vi "Main.vi"(8 "error in":errorcluster, 11 "TCP Read in":refnum<class "TCP Read.lvclass">) -> (0 "error out":errorcluster, 3 "TCP Read out":refnum<class "TCP Read.lvclass">)   [LabVIEW 2017, in "_TCP Client.lvlib" / "TCP Read.lvclass"]
doc: "The <b>Queued Message Handler</b> of the Worker that owns this VI."
uses:
  TCP Read.lvclass
  C:/SC/Source Code/VIPM/LabVIEW 20xx/vi.lib/addons/_Workers/Library/Classes/Worker/Worker.lvclass
  Initialization Data.ctl
  Response Cases.ctl
  <vilib>/addons/_Workers/Library/Case Label.ctl
  <vilib>/addons/_Workers/Library/Classes/Message Queue/Message Queue.lvclass
  TCP Read.lvclass/TCP Read.ctl
  rsp_Connection Lost.ctl
  <vilib>/addons/_Workers/Library/Workers.lvlib
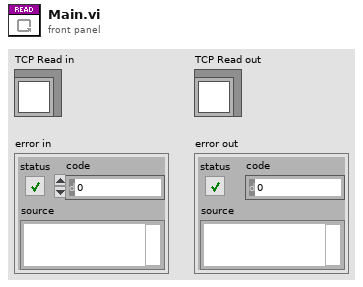
[diagram p1: front panel]
types:
  T1 = typedef "_TCP Client.lvlib/TCP Read.lvclass/Initialization Data.ctl" = cluster{"Response Cases":T2, "Connection ID":refnum<k5>, "Forwarding Queue":refnum<class "Message Queue.lvclass">, "Forwarding Case":T3, "Server Name":string}
  T2 = typedef "_TCP Client.lvlib/TCP Read.lvclass/Response Cases.ctl" = cluster{"Connection Lost":T3}
  T3 = typedef "Workers.lvlib/Case Label.ctl" = string
  T4 = enum16{"Standard", "Buffered", "CRLF", "Immediate"}
  T5 = typedef "_TCP Client.lvlib/TCP Read.lvclass/rsp_Connection Lost.ctl" = cluster{"Connection ID":refnum<k5>, "TCP Read Queue":refnum<class "Message Queue.lvclass">}
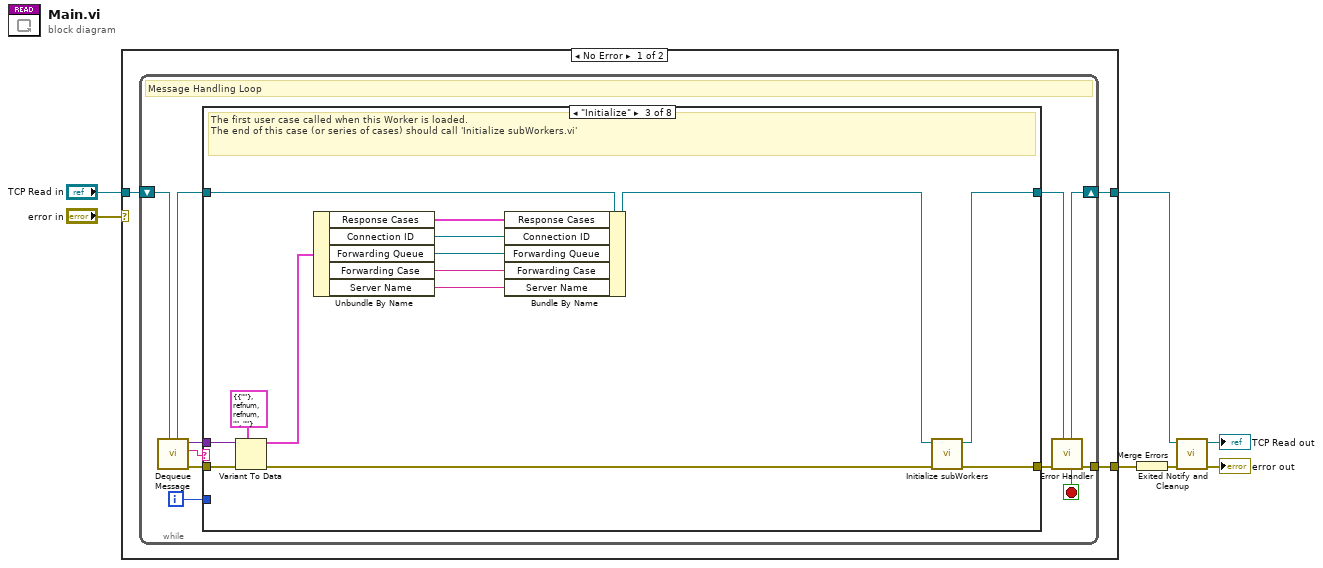
[diagram p0: block diagram]
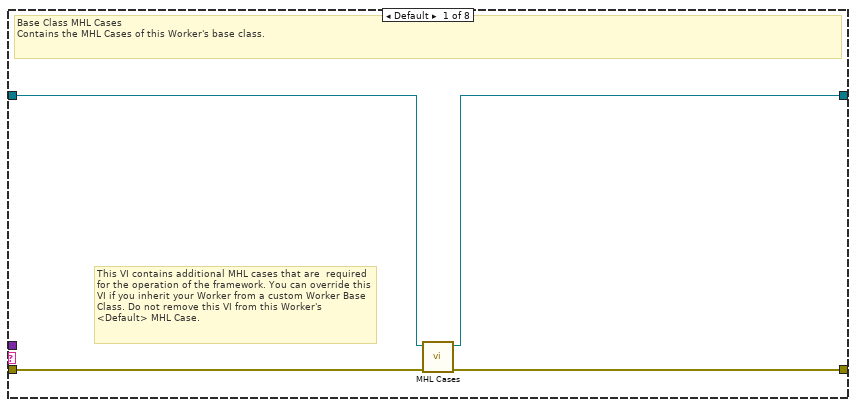
[diagram p2: hidden frame]
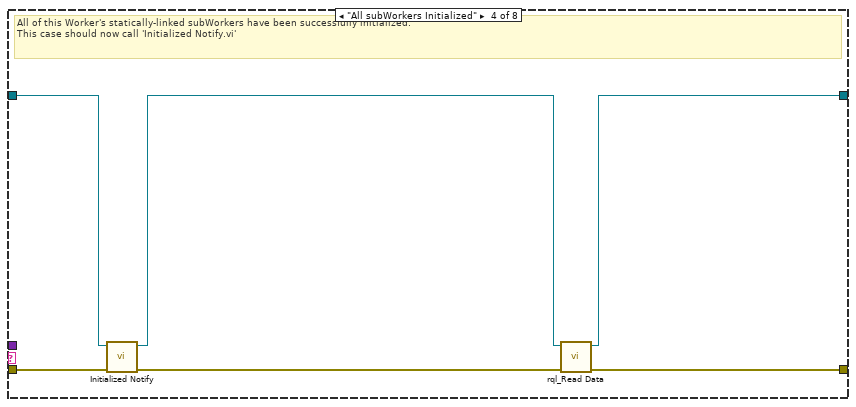
[diagram p4: hidden frame]
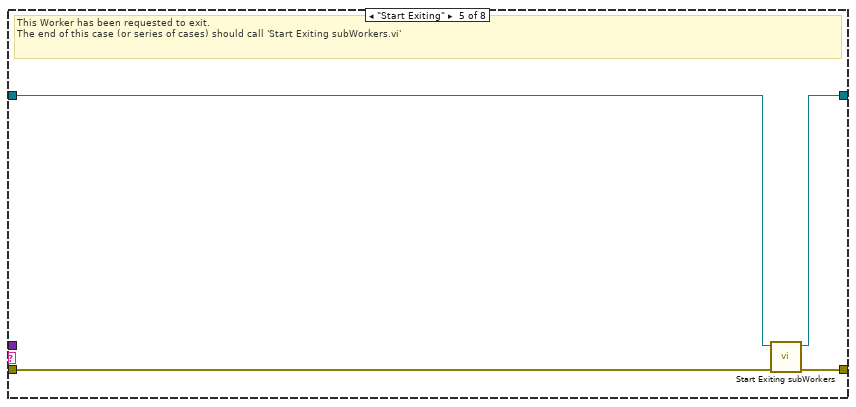
[diagram p5: hidden frame]
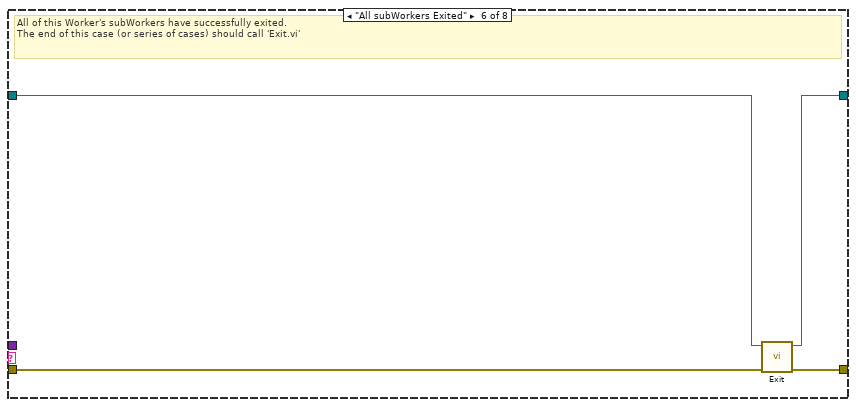
[diagram p6: hidden frame]
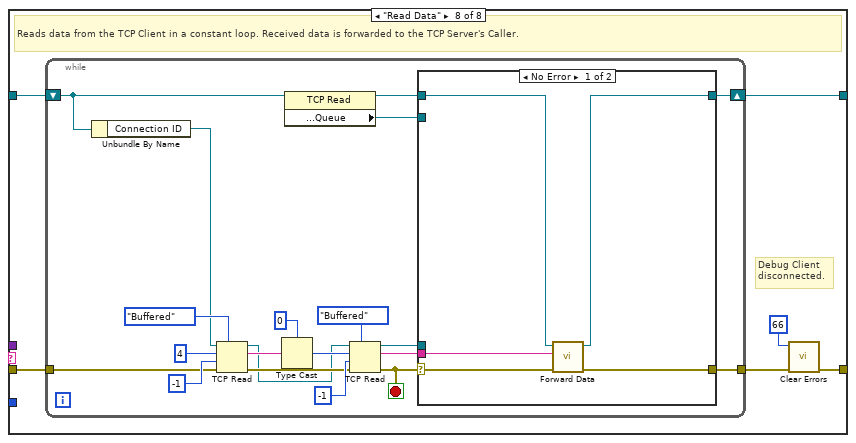
[diagram p8: hidden frame]
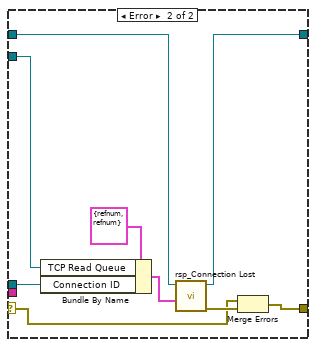
[diagram p9: hidden frame]
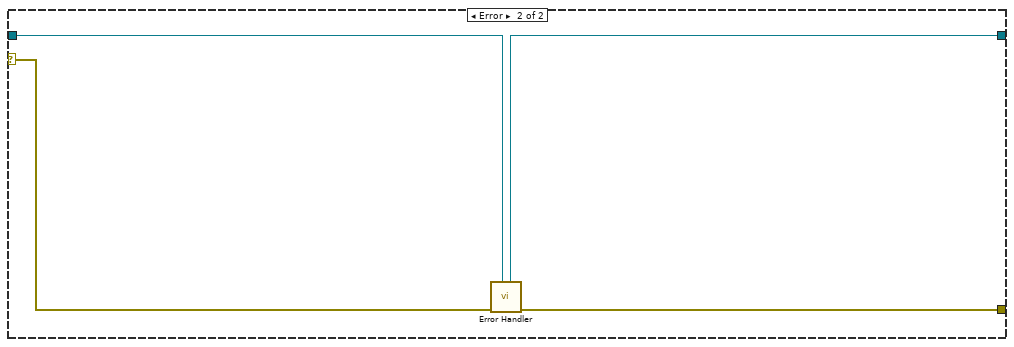
[diagram p10: hidden frame]
diagram:
  n1 = case shown="No Error" "error in" {
    tunnel: "TCP Read in" -> [w8 w99]
    tunnel: [w10 w100] -> w1
    tunnel: [w9 w98] -> w7
    selector: "error in" -> [_ w101]
    frame No Error {
      n2 = while {
        shift-right: [w19] -> w9
        shift-left: w8 -> [w21]
        tunnel: [w20] -> w10
        i -> [w12]
        stop <- w13 stop-if-true
        # "Message Handling Loop"
        n3 = call-dynamic "Dequeue Message.vi"("Worker"=w21) -> ("error out"=w18:errorcluster, "Case out"=w14:string, "Data out"=w11:variant, "Worker out"=w16:refnum<class "TCP Read.lvclass">)  [unwired: 6 in, 1 out]
        n4 = case "Worker MHL Case Structure (DO NOT CHANGE LABEL NAME)" shown="\"Initialize\"" w14 {
          tunnel: w18 -> [w25 w26 w39 w47 w48 w55 w57 w61]
          tunnel: [w24 w26 w41 w44 w51 w54 w57 w58] -> w17
          tunnel: w16 -> [w23 w27 w38 w45 w49 w53 w56 w62]
          tunnel: [w22 w27 w40 w42 w50 w52 w56 w63] -> w15
          tunnel: w12 -> [_ _ _ _ _ _ _ _]
          tunnel: w11 -> [_ _ w36 _ _ _ _ _]
          frame Default {
            # "This VI contains additional MHL cases that are  required for the operation of the framework. You can override this VI if you inherit your Worker from a custom Worker Base Class. Do not remove this VI from this Worker's <Default> MHL Case."
            # "Base Class MHL Cases\nContains the MHL Cases of this Worker's base class."
            n5 = call-dynamic "MHL Cases.vi"("error in"=w25, "Worker in"=w23) -> ("error out"=w24:errorcluster, "Worker out"=w22:refnum<class "TCP Read.lvclass">)  [unwired: 8 in]
          }
          frame "------------ FRAMEWORK CASES -----------" {
            # "Start of Workers Framework Cases"
          }
          frame "Initialize" {
            # "The first user case called when this Worker is loaded.\nThe end of this case (or series of cases) should call 'Initialize subWorkers.vi'"
            n6 = Variant To Data(error in=w39, type=T1 {"Response Cases"={"Connection Lost"=""}, "Connection ID"=refnum, "Forwarding Queue"=refnum, "Forwarding Case"="", "Server Name"=""} ("Cluster"), Variant=w36) -> (data=w34:T1, error out=w37:errorcluster)
            n7 = Unbundle By Name(w34) -> ("Response Cases"=w33:T2, "Connection ID"=w31:refnum<k5>, "Forwarding Queue"=w30:refnum<class "Message Queue.lvclass">, "Forwarding Case"=w29:T3, "Server Name"=w28:string)
            n8 = Bundle By Name(cluster=w38, "Response Cases"=w33, "Connection ID"=w31, "Forwarding Queue"=w30, "Forwarding Case"=w29, "Server Name"=w28) -> (w35:refnum<class "TCP Read.lvclass">)
            n9 = call-dynamic "Initialize subWorkers.vi"("error in"=w37, "Worker"=w35) -> ("error out"=w41:errorcluster, "dup Worker out"=w40:refnum<class "TCP Read.lvclass">)  [unwired: 8 in]
          }
          frame "All subWorkers Initialized" {
            # "All of this Worker's statically-linked subWorkers have been successfully initialized.\nThis case should now call 'Initialized Notify.vi'"
            n10 = call-dynamic "Initialized Notify.vi"("error in"=w47, "Worker"=w45) -> ("error out"=w46:errorcluster, "dup Worker out"=w43:refnum<class "TCP Read.lvclass">)  [unwired: 8 in]
            n11 = call "rql_Read Data.vi"("error in"=w46, "TCP Read in"=w43) -> ("error out"=w44:errorcluster, "dup TCP Read out"=w42:refnum<class "TCP Read.lvclass">)  [unwired: 8 in]
          }
          frame "Start Exiting" {
            # "This Worker has been requested to exit. \nThe end of this case (or series of cases) should call 'Start Exiting subWorkers.vi'"
            n12 = call-dynamic "Start Exiting subWorkers.vi"("error_in"=w48, "Worker"=w49) -> ("error out"=w51:errorcluster, "dup Worker out"=w50:refnum<class "TCP Read.lvclass">)  [unwired: 8 in]
          }
          frame "All subWorkers Exited" {
            # "All of this Worker's subWorkers have successfully exited. \nThe end of this case (or series of cases) should call 'Exit.vi'"
            n13 = call-dynamic "Exit.vi"("error_in"=w55, "Worker"=w53) -> ("error out"=w54:errorcluster, "dup Worker out"=w52:refnum<class "TCP Read.lvclass">)  [unwired: 8 in]
          }
          frame "------------- LOCAL API CASES -------------" {
            # "Start of Workers Local API Cases"
          }
          frame "Read Data" {
            # "Debug Client\ndisconnected."
            # "Reads data from the TCP Client in a constant loop. Received data is forwarded to the TCP Server's Caller."
            n14 = while {
              shift-right: [w82] -> w63
              shift-left: w62 -> [w70]
              tunnel: [w83] -> w59
              tunnel: w61 -> [w71]
              stop <- w68 stop-if-true
              n15 = Unbundle By Name(w70) -> ("Connection ID"=w69:refnum<k5>)
              n16 = TCP Read(connection ID=w69, bytes to read=4, error in (no error)=w71, 7:T4."Buffered" ("mode (standard)"), 9:-1 ("timeout ms (25000)")) -> (connection ID out=w72:refnum<k5>, data out=w73:string, error out=w74:errorcluster)
              n17 = Type Cast(type=0 ("bytes to read"), x=w73) -> (*(type *) &x=w76:i32)
              n18 = property class="TCP Read"(reference=w70) -> (reference out=w65:refnum<class "TCP Read.lvclass">, "Accessors:Read:Public API:Queue"=w64:refnum<class "Message Queue.lvclass">)  [unwired: 1 in, 1 out]
              n19 = TCP Read(connection ID=w72, bytes to read=w76, error in (no error)=w74, 7:T4."Buffered" ("mode (standard)"), 9:-1 ("timeout ms (25000)")) -> (connection ID out=w66:refnum<k5>, data out=w67:string, error out=w68:errorcluster)
              n20 = case shown="No Error" w68 {
                selector: w68 -> [w87 w93]
                tunnel: [w88 w94] -> w83
                tunnel: [w85 w96] -> w82
                tunnel: w65 -> [w86 w95]
                tunnel: w67 -> [w84 _]
                tunnel: w66 -> [_ w90]
                tunnel: w64 -> [_ w89]
                frame No Error {
                  n21 = call "Forward Data.vi"("error in (no error)"=w87, "Data"=w84, "TCP Read in"=w86) -> ("error out"=w88:errorcluster, "TCP Read out"=w85:refnum<class "TCP Read.lvclass">)  [unwired: 7 in]
                }
                frame Error {
                  n22 = Bundle By Name(cluster=T5 {"Connection ID"=refnum, "TCP Read Queue"=refnum} ("Data in"), "TCP Read Queue"=w89, "Connection ID"=w90) -> (w91:T5)
                  n23 = call "rsp_Connection Lost.vi"("Data in"=w91, "TCP Read in"=w95) -> ("error out"=w97:errorcluster, "dup TCP Read out"=w96:refnum<class "TCP Read.lvclass">)  [unwired: 8 in]
                  n24 = Merge Errors(w93, w97) -> (w94:errorcluster)
                }
              }
            }
            n25 = call <vilib>:"Clear Errors.vi"("error in (no error)"=w59, "specific error code to clear (0: all)"=66) -> ("error out"=w58:errorcluster)  [unwired: 4 in, 1 out]
          }
        }
        n26 = call-dynamic "Error Handler.vi"("Worker"=w15, "error_in"=w17) -> ("error out"=w20:errorcluster, "Stop Loop"=w13:bool, "Worker out"=w19:refnum<class "TCP Read.lvclass">)  [unwired: 7 in]
      }
    }
    frame Error {
      n27 = call-dynamic "Error Handler.vi"("Worker"=w99, "error_in"=w101) -> ("error out"=w100:errorcluster, "Worker out"=w98:refnum<class "TCP Read.lvclass">)  [unwired: 7 in, 1 out]
    }
  }
  n28 = Merge Errors(w1) -> (w4:errorcluster)
  n29 = call-dynamic "Exited Notify and Cleanup.vi"("error_in"=w4, "Worker"=w7) -> ("error out"=→"error out":errorcluster, "dup Worker out"=→"TCP Read out":refnum<class "TCP Read.lvclass">)  [unwired: 8 in]
